vi "Remove and Rewire.vi"(6 "Variant in":variant caption="变体输入", 7 "Shift Pressed?":bool caption="按下Shift？", 8 "error in (no error)":errorcluster caption="错误输入（无错误）", 10 "QD Combo Box Ref":refnum<vi> caption="快速放置组合框引用", 11 "QD Launch VI Ref":refnum<vi> caption="快速放置启动VI引用") -> (0 "error out":errorcluster caption="错误输出", 4 "Variant out":variant caption="变体输出")   [LabVIEW 2016]
doc: "删除所选程序框图对象和与之相连的全部控件和常量，并在被删除对象数据类型相同的输入输出接线端之间连线。\n\n默认快捷键 - [R]"
panel:
  in  "Undo Name":string="快速放置删除" caption="撤消名称"
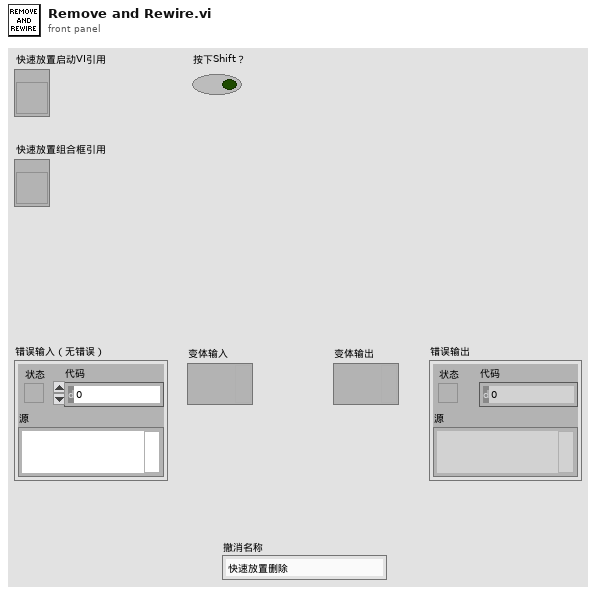
[diagram p1: front panel]
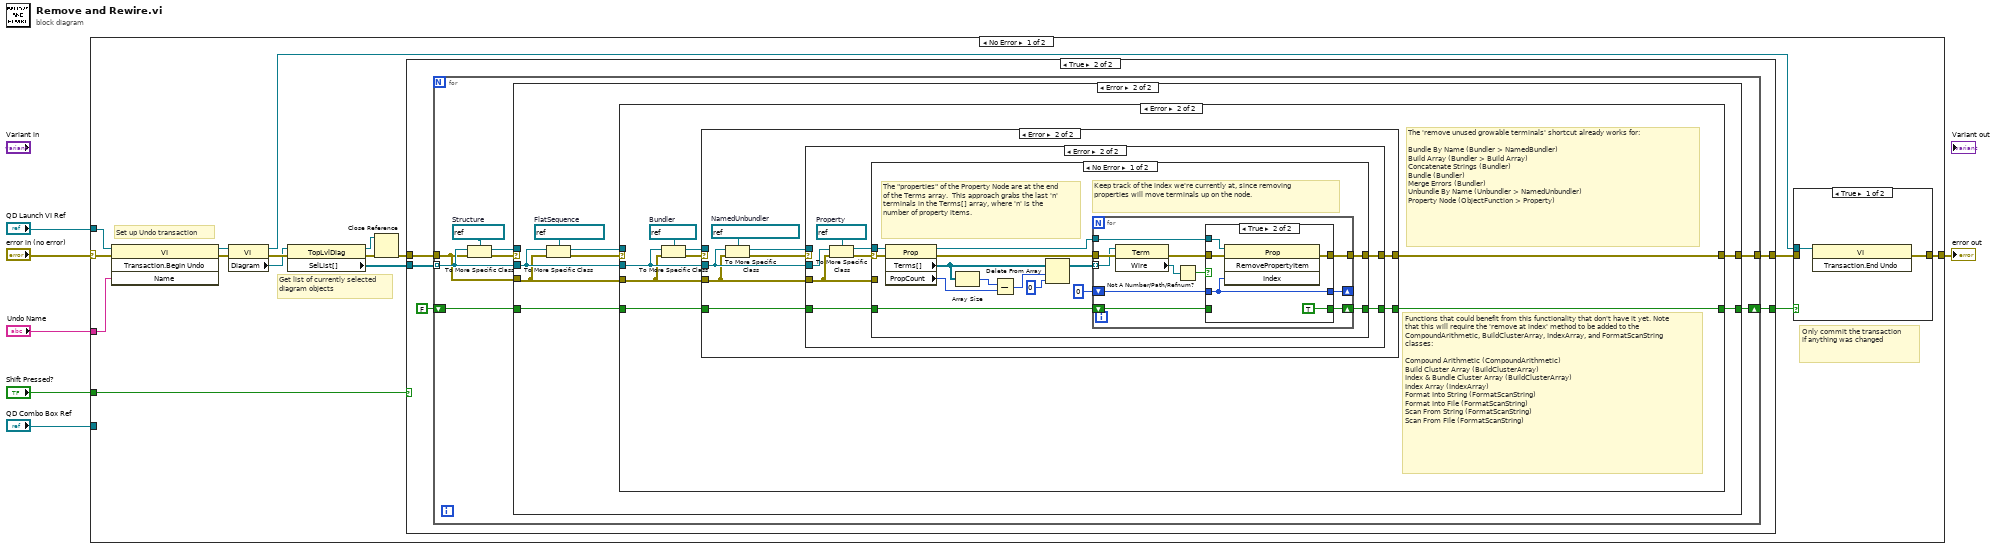
[diagram p0: block diagram]
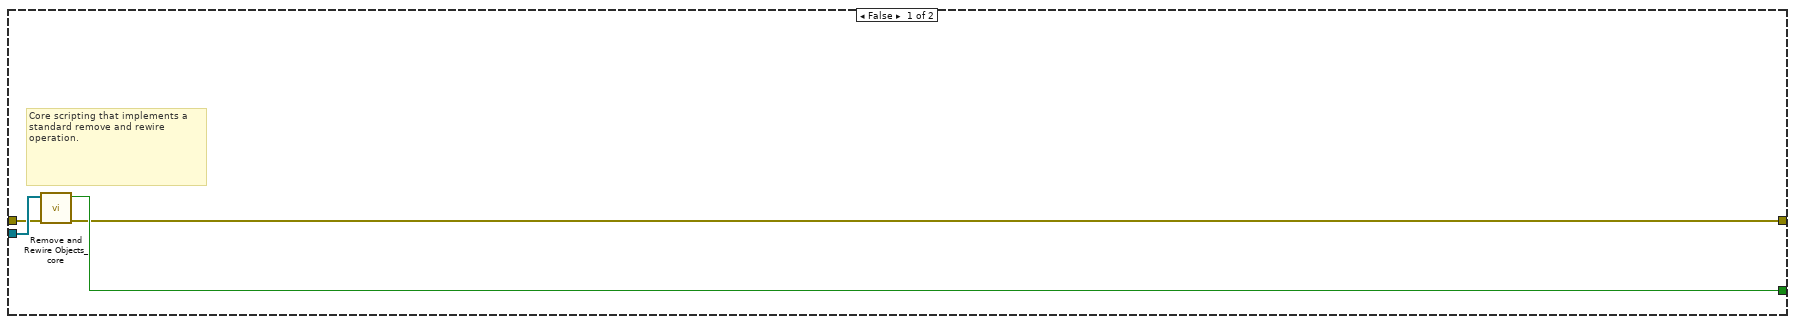
[diagram p2: hidden frame]
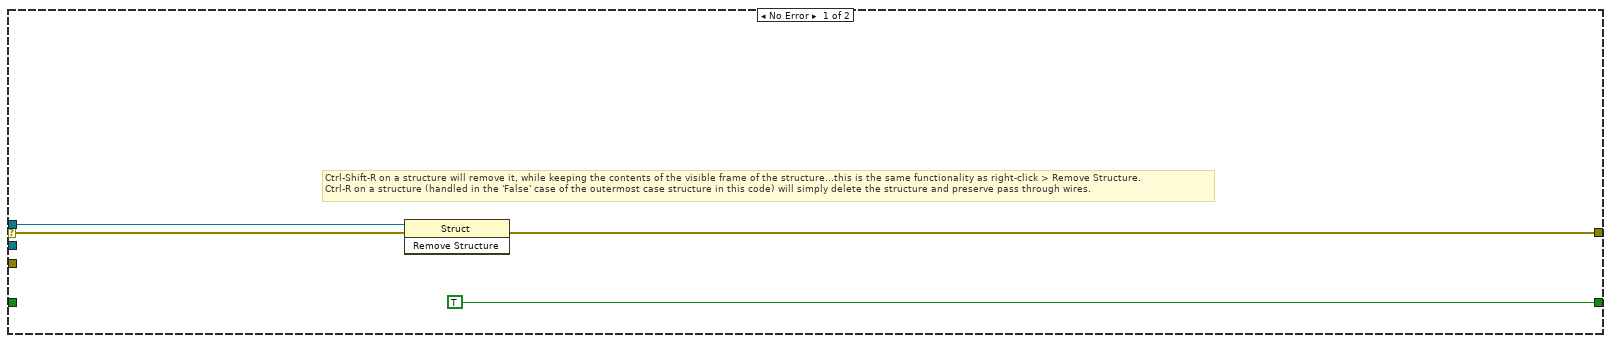
[diagram p3: hidden frame]
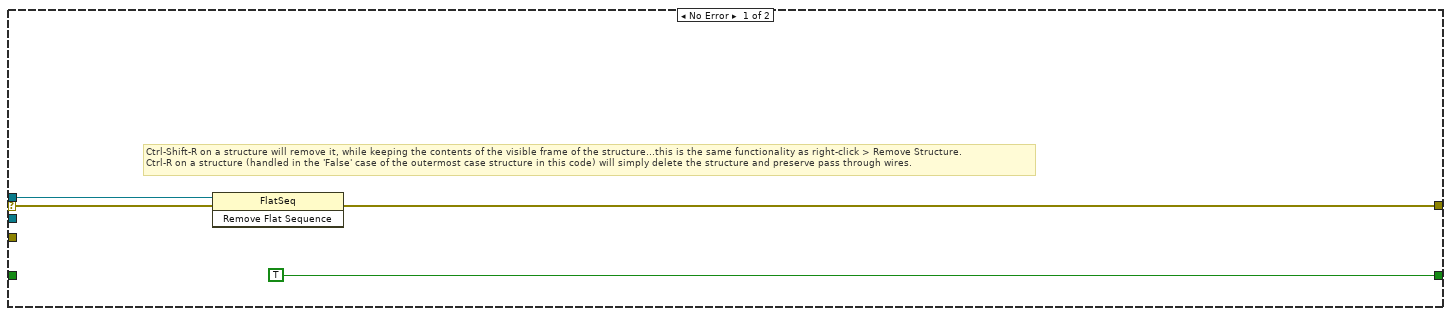
[diagram p4: hidden frame]
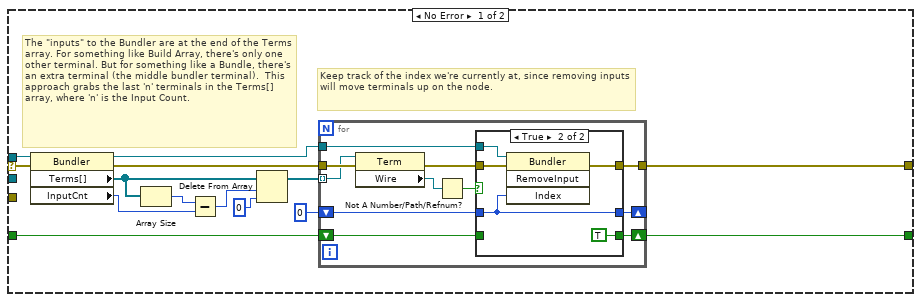
[diagram p5: hidden frame]
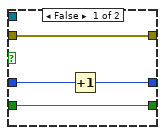
[diagram p6: hidden frame]
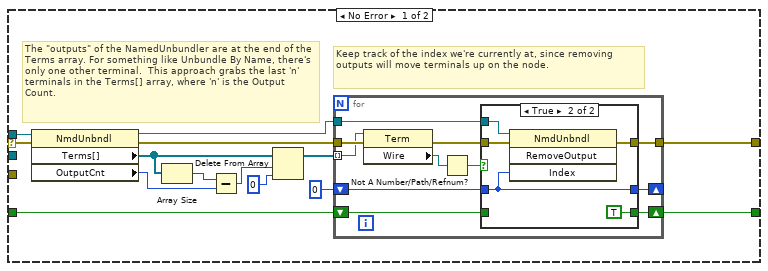
[diagram p7: hidden frame]
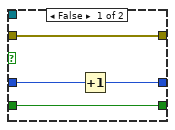
[diagram p8: hidden frame]
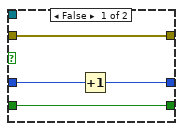
[diagram p9: hidden frame]
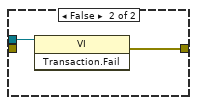
[diagram p11: hidden frame]
diagram:
  n1 = case shown="No Error" "error in (no error)" {
    selector: "error in (no error)" -> [w12 w188]
    tunnel: [w10 w188] -> w5
    tunnel: "QD Launch VI Ref" -> [w11 _]
    tunnel: "Shift Pressed?" -> [w9 _]
    tunnel: "QD Combo Box Ref" -> [_ _]
    tunnel: "Undo Name" -> [w7 _]
    frame No Error {
      # "Get list of currently selected\ndiagram objects"
      # "Set up Undo transaction"
      # "Only commit the transaction\nif anything was changed"
      n2 = invoke class="VI" method="Transaction.Begin Undo"(reference=w11, error in=w12, "Name"=w7) -> (reference out=w17:refnum<vi>, error out=w18:errorcluster)  [unwired: 1 in, 2 out]
      n3 = property class="VI"(reference=w17, error in=w18) -> (reference out=w15:refnum<vi>, error out=w22:errorcluster, "Diagram"=w21:refnum<vi>)
      n4 = property class="TopLvlDiag"(reference=w21, error in=w22) -> (reference out=w19:refnum<vi>, error out=w20:errorcluster, "SelList[]"=w16:refnum<vi>[])
      n5 = Close Reference(reference=w19, error in (no error)=w20) -> (error out=w13:errorcluster)
      n6 = case shown="True" w9 {
        tunnel: w16 -> [w24 w30]
        tunnel: [w26 w28] -> w14
        tunnel: w13 -> [w23 w31]
        tunnel: [w25 w29] -> w8
        frame False {
          # "Core scripting that implements a standard remove and rewire operation."
          n7 = call <vilib>:"Remove and Rewire Objects_core.vi"("error in (no error)"=w23, "Items to Remove"=w24) -> ("error out"=w25:errorcluster, "Any Items Removed?"=w26:bool)  [unwired: 8 in]
        }
        frame True {
          n8 = for {
            tunnel: w30 -> [w36] mode=indexing
            shift-right: [w37] -> w28
            shift-left: FALSE -> [w38]
            tunnel: w31 -> [w33]
            tunnel: [w39] -> w29
            w35 = refnum<vi> refnum  # Structure
            n9 = To More Specific Class(target class=w35, reference=w36, error in=w33) -> (specific class reference=w32:refnum<vi>, error out=w34:errorcluster)
            n10 = case shown="Error" w34 {
              selector: w34 -> [w43 _]
              tunnel: [w41 w51] -> w39
              tunnel: w38 -> [_ w50]
              tunnel: [TRUE w49] -> w37
              tunnel: w36 -> [_ w47]
              tunnel: w33 -> [_ w46]
              tunnel: w32 -> [w42 _]
              frame No Error {
                # "Ctrl-Shift-R on a structure will remove it, while keeping the contents of the visible frame of the structure...this is the same functionality as right-click > Remove Structure.\nCtrl-R on a structure (handled in the 'False' case of the outermost case structure in this code) will simply delete the structure and preserve pass through wires."
                n11 = invoke class="Struct" method="Remove Structure"(reference=w42, error in=w43) -> (error out=w41:errorcluster)  [unwired: 1 in, 2 out]
              }
              frame Error {
                w48 = refnum<vi> refnum  # FlatSequence
                n12 = To More Specific Class(target class=w48, reference=w47, error in=w46) -> (specific class reference=w44:refnum<vi>, error out=w45:errorcluster)
                n13 = case shown="Error" w45 {
                  selector: w45 -> [w54 _]
                  tunnel: [w52 w60] -> w51
                  tunnel: w50 -> [_ w59]
                  tunnel: [TRUE w58] -> w49
                  tunnel: w47 -> [_ w57]
                  tunnel: w46 -> [_ w56]
                  tunnel: w44 -> [w55 _]
                  frame No Error {
                    # "Ctrl-Shift-R on a structure will remove it, while keeping the contents of the visible frame of the structure...this is the same functionality as right-click > Remove Structure.\nCtrl-R on a structure (handled in the 'False' case of the outermost case structure in this code) will simply delete the structure and preserve pass through wires."
                    n14 = invoke class="FlatSeq" method="Remove Flat Sequence"(reference=w55, error in=w54) -> (error out=w52:errorcluster)  [unwired: 1 in, 2 out]
                  }
                  frame Error {
                    w63 = refnum<vi> refnum  # Bundler
                    # "Functions that could benefit from this functionality that don't have it yet. Note that this will require the 'remove at index' method to be added to the CompoundArithmetic, BuildClusterArray, IndexArray, and FormatScanString classes:\n\nCompound Arithmetic (CompoundArithmetic)\nBuild Cluster Array (BuildClusterArray)\nIndex & Bundle Cluster Array (BuildClusterArray)\nIndex Array (IndexArray)\nFormat Into String (FormatScanString)\nFormat Into File (FormatScanString)\nScan From String (FormatScanString)\nScan From File (FormatScanString)"
                    # "The 'remove unused growable terminals' shortcut already works for:\n\nBundle By Name (Bundler > NamedBundler)\nBuild Array (Bundler > Build Array)\nConcatenate Strings (Bundler)\nBundle (Bundler)\nMerge Errors (Bundler)\nUnbundle By Name (Unbundler > NamedUnbundler)\nProperty Node (ObjectFunction > Property)"
                    n15 = To More Specific Class(target class=w63, reference=w57, error in=w56) -> (specific class reference=w61:refnum<vi>, error out=w62:errorcluster)
                    n16 = case shown="Error" w62 {
                      selector: w62 -> [w64 _]
                      tunnel: w61 -> [w65 _]
                      tunnel: w57 -> [_ w99]
                      tunnel: w56 -> [_ w98]
                      tunnel: [w77 w105] -> w60
                      tunnel: w59 -> [w76 w104]
                      tunnel: [w75 w103] -> w58
                      frame No Error {
                        # "Keep track of the index we're currently at, since removing inputs will move terminals up on the node."
                        # "The \"inputs\" to the Bundler are at the end of the Terms array. For something like Build Array, there's only one other terminal. But for something like a Bundle, there's an extra terminal (the middle bundler terminal).  This approach grabs the last 'n' terminals in the Terms[] array, where 'n' is the Input Count."
                        n17 = property class="Bundler"(reference=w65, error in=w64) -> (reference out=w71:refnum<vi>, error out=w74:errorcluster, "Terms[]"=w69:refnum<vi>[], "InputCnt"=w67:i32)
                        n18 = Array Size(array=w69) -> (size(s)=w68:i32)
                        n19 = Subtract(x=w68, y=w67) -> (x-y=w66:i32)
                        n20 = Delete From Array(array=w69, length=w66, index=0) -> (array with subset deleted=w73:refnum<vi>[])  [unwired: 1 out]
                        n21 = for {
                          tunnel: w73 -> [w87] mode=indexing
                          shift-right: [w79] -> _
                          shift-left: 0 -> [w83]
                          shift-right: [w80] -> w75
                          shift-left: w76 -> [w82]
                          tunnel: w71 -> [w78]
                          tunnel: w74 -> [w88]
                          tunnel: [w81] -> w77
                          n22 = property class="Term"(reference=w87, error in=w88) -> (error out=w84:errorcluster, "Wire"=w86:refnum<vi>)  [unwired: 1 out]
                          n23 = Not A Number/Path/Refnum?(number/path/refnum=w86) -> (NaN/Path/Refnum?=w85:bool)
                          n24 = case shown="True" w85 {
                            tunnel: w84 -> [w92 w96]
                            tunnel: w83 -> [w90 w93]
                            tunnel: w82 -> [w91 _]
                            tunnel: [w92 w94] -> w81
                            tunnel: [w91 TRUE] -> w80
                            tunnel: [w89 w93] -> w79
                            tunnel: w78 -> [_ w95]
                            frame False {
                              n25 = Increment(x=w90) -> (x+1=w89:i32)
                            }
                            frame True {
                              n26 = invoke class="Bundler" method="RemoveInput"(reference=w95, error in=w96, "Index"=w93) -> (error out=w94:errorcluster)  [unwired: 1 in, 3 out]
                            }
                          }
                        }
                      }
                      frame Error {
                        w101 = refnum<vi> refnum  # NamedUnbundler
                        n27 = To More Specific Class(target class=w101, reference=w99, error in=w98) -> (specific class reference=w102:refnum<vi>, error out=w100:errorcluster)
                        n28 = case shown="Error" w100 {
                          selector: w100 -> [w106 _]
                          tunnel: [w119 w147] -> w105
                          tunnel: w104 -> [w118 w146]
                          tunnel: [w117 w145] -> w103
                          tunnel: w102 -> [w107 _]
                          tunnel: w99 -> [_ w142]
                          tunnel: w98 -> [_ w140]
                          frame No Error {
                            # "Keep track of the index we're currently at, since removing outputs will move terminals up on the node."
                            # "The \"outputs\" of the NamedUnbundler are at the end of the Terms array. For something like Unbundle By Name, there's only one other terminal.  This approach grabs the last 'n' terminals in the Terms[] array, where 'n' is the Output Count."
                            n29 = property class="NmdUnbndl"(reference=w107, error in=w106) -> (reference out=w113:refnum<vi>, error out=w116:errorcluster, "Terms[]"=w108:refnum<vi>[], "OutputCnt"=w110:i32)
                            n30 = Array Size(array=w108) -> (size(s)=w111:i32)
                            n31 = Subtract(x=w111, y=w110) -> (x-y=w109:i32)
                            n32 = Delete From Array(array=w108, length=w109, index=0) -> (array with subset deleted=w115:refnum<vi>[])  [unwired: 1 out]
                            n33 = for {
                              tunnel: w115 -> [w129] mode=indexing
                              shift-right: [w121] -> _
                              shift-left: 0 -> [w125]
                              shift-right: [w122] -> w117
                              shift-left: w118 -> [w124]
                              tunnel: w113 -> [w120]
                              tunnel: w116 -> [w130]
                              tunnel: [w123] -> w119
                              n34 = property class="Term"(reference=w129, error in=w130) -> (error out=w126:errorcluster, "Wire"=w128:refnum<vi>)  [unwired: 1 out]
                              n35 = Not A Number/Path/Refnum?(number/path/refnum=w128) -> (NaN/Path/Refnum?=w127:bool)
                              n36 = case shown="True" w127 {
                                tunnel: w126 -> [w134 w138]
                                tunnel: w125 -> [w132 w135]
                                tunnel: w124 -> [w133 _]
                                tunnel: [w134 w136] -> w123
                                tunnel: [w133 TRUE] -> w122
                                tunnel: [w131 w135] -> w121
                                tunnel: w120 -> [_ w137]
                                frame False {
                                n37 = Increment(x=w132) -> (x+1=w131:i32)
                                }
                                frame True {
                                n38 = invoke class="NmdUnbndl" method="RemoveOutput"(reference=w137, error in=w138, "Index"=w135) -> (error out=w136:errorcluster)  [unwired: 1 in, 3 out]
                                }
                              }
                            }
                          }
                          frame Error {
                            w143 = refnum<vi> refnum  # Property
                            n39 = To More Specific Class(target class=w143, reference=w142, error in=w140) -> (specific class reference=w144:refnum<vi>, error out=w141:errorcluster)
                            n40 = case shown="No Error" w141 {
                              selector: w141 -> [w148 _]
                              tunnel: [w161 w183] -> w147
                              tunnel: w146 -> [w160 w182]
                              tunnel: [w159 w182] -> w145
                              tunnel: w144 -> [w149 _]
                              tunnel: w140 -> [_ w183]
                              frame No Error {
                                # "Keep track of the index we're currently at, since removing properties will move terminals up on the node."
                                # "The \"properties\" of the Property Node are at the end of the Terms array.  This approach grabs the last 'n' terminals in the Terms[] array, where 'n' is the number of property items."
                                n41 = property class="Prop"(reference=w149, error in=w148) -> (reference out=w155:refnum<vi>, error out=w158:errorcluster, "Terms[]"=w150:refnum<vi>[], "PropCount"=w152:i32)
                                n42 = Array Size(array=w150) -> (size(s)=w153:i32)
                                n43 = Subtract(x=w153, y=w152) -> (x-y=w151:i32)
                                n44 = Delete From Array(array=w150, length=w151, index=0) -> (array with subset deleted=w157:refnum<vi>[])  [unwired: 1 out]
                                n45 = for {
                                tunnel: w157 -> [w171] mode=indexing
                                shift-right: [w163] -> _
                                shift-left: 0 -> [w167]
                                shift-right: [w164] -> w159
                                shift-left: w160 -> [w166]
                                tunnel: w155 -> [w162]
                                tunnel: w158 -> [w172]
                                tunnel: [w165] -> w161
                                n46 = property class="Term"(reference=w171, error in=w172) -> (error out=w168:errorcluster, "Wire"=w170:refnum<vi>)  [unwired: 1 out]
                                n47 = Not A Number/Path/Refnum?(number/path/refnum=w170) -> (NaN/Path/Refnum?=w169:bool)
                                n48 = case shown="True" w169 {
                                tunnel: w168 -> [w176 w180]
                                tunnel: w167 -> [w174 w177]
                                tunnel: w166 -> [w175 _]
                                tunnel: [w176 w178] -> w165
                                tunnel: [w175 TRUE] -> w164
                                tunnel: [w173 w177] -> w163
                                tunnel: w162 -> [_ w179]
                                frame False {
                                n49 = Increment(x=w174) -> (x+1=w173:i32)
                                }
                                frame True {
                                n50 = invoke class="Prop" method="RemovePropertyItem"(reference=w179, error in=w180, "Index"=w177) -> (error out=w178:errorcluster)  [unwired: 1 in, 3 out]
                                }
                                }
                                }
                              }
                              frame Error {
                                # "This is not a supported GrowableFunction.  The Ctrl-Shift-R shortcut does not apply."
                              }
                            }
                          }
                        }
                      }
                    }
                  }
                }
              }
            }
          }
        }
      }
      n51 = case shown="True" w14 {
        tunnel: w15 -> [w184 w186]
        tunnel: [w185 w187] -> w10
        tunnel: w8 -> [_ _]
        frame True {
          n52 = invoke class="VI" method="Transaction.End Undo"(reference=w184) -> (error out=w185:errorcluster)  [unwired: 2 in, 2 out]
        }
        frame False {
          n53 = invoke class="VI" method="Transaction.Fail"(reference=w186) -> (error out=w187:errorcluster)  [unwired: 2 in, 2 out]
        }
      }
    }
    frame Error {
    }
  }
  "error out" <- w5
